vi "DATADYNTEST.vi"(8 "errin":errorcluster, 9 "SN":string="0B5MEVA000CA1JC1M0000041", 10 "Limites":T1, 11 "visain":refnum<visa-resource-name>) -> (0 "errout":errorcluster, 2 "chaîne concaténée":string, 3 "visaout":refnum<visa-resource-name>)   [LabVIEW 2020]
doc: "Test et trace en BDD l'OCV et les V/TCell"
uses:
  <vilib>/addons/database/Connection.llb/DB Tools Open Connec (String).vi
  <vilib>/addons/database/Connection.llb/Conn Execute.vi
  <vilib>/addons/database/Recordset.llb/Rec Destroy - Connection.vi
  <vilib>/addons/database/NI_Database_API.lvlib
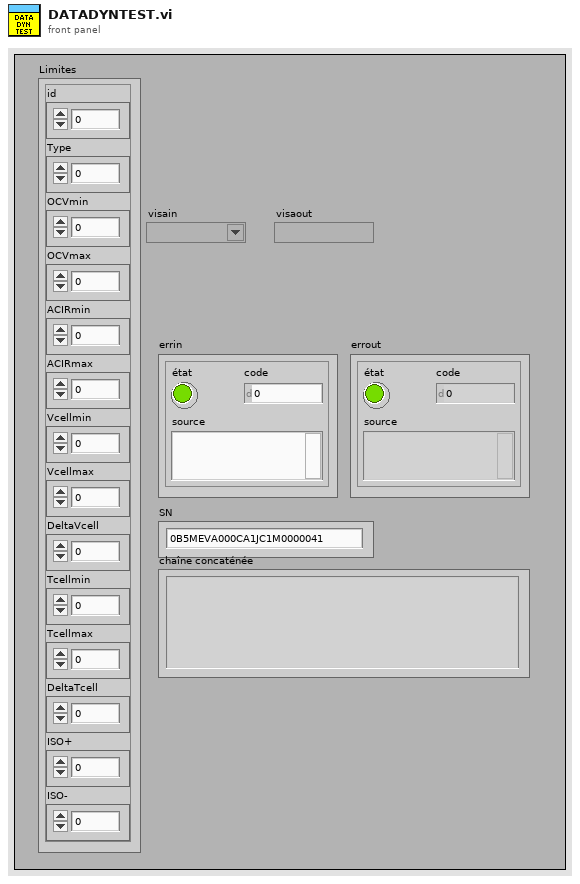
[diagram p1: front panel]
types:
  T1 = cluster{"id":dbl, "Type":dbl, "OCVmin":dbl, "OCVmax":dbl, "ACIRmin":dbl, "ACIRmax":dbl, "Vcellmin":dbl, "Vcellmax":dbl, "DeltaVcell":dbl, "Tcellmin":dbl, "Tcellmax":dbl, "DeltaTcell":dbl, "ISO+":dbl, "ISO-":dbl}
  T2 = cluster{"Cell1 V":sgl, "Cell2 V":sgl, "Cell3 V":sgl, "Cell4 V":sgl, "Cell1 °C":sgl, "Cell2 °C":sgl, "Cell5 V":sgl, "Cell6 V":sgl}
  T3 = typedef "NI_Database_API.lvlib/Conn ObjectReference.ctl" = refnum<k1>
  T4 = typedef "NI_Database_API.lvlib/Rec ObjectReference.ctl" = refnum<k1>
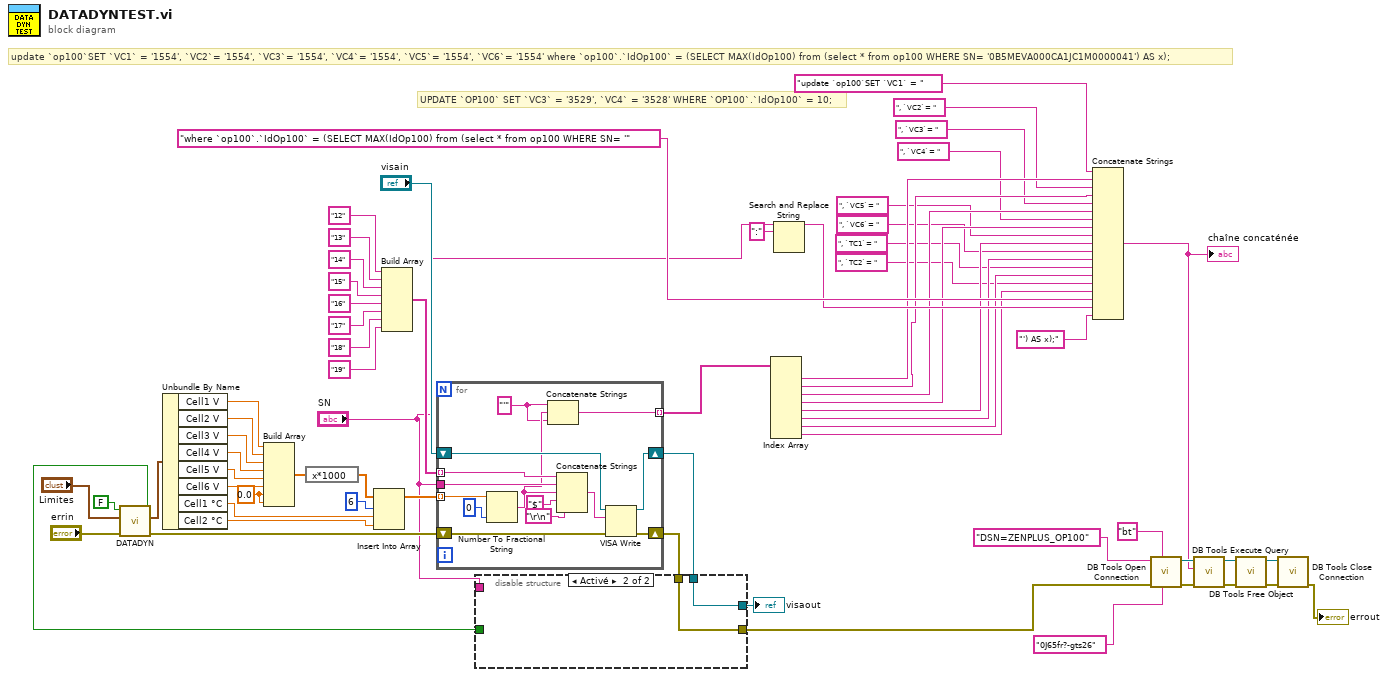
[diagram p0: block diagram]
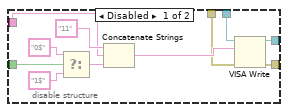
[diagram p2: hidden frame]
diagram:
  w39 = sgl 0.0 ("élément")
  # "update `op100`SET `VC1` = '1554', `VC2`= '1554', `VC3`= '1554', `VC4`= '1554', `VC5`= '1554', `VC6`= '1554' where `op100`.`IdOp100` = (SELECT MAX(IdOp100) from (select * from op100 WHERE SN= '0B5MEVA000CA1JC1M0000041') AS x);"
  # "UPDATE `OP100` SET `VC3` = '3529', `VC4` = '3528' WHERE `OP100`.`IdOp100` = 10;"
  n1 = call "DATADYN.vi"("errin"="errin", "Limites"="Limites", "3P4S"=FALSE) -> ("errout"=w64:errorcluster, "Out"=w42:T2, "test OK?"=w38:bool)  [unwired: 5 in, 1 out]
  n2 = Unbundle By Name(w42) -> ("Cell1 V"=w52:sgl, "Cell2 V"=w53:sgl, "Cell3 V"=w54:sgl, "Cell4 V"=w55:sgl, "Cell5 V"=w56:sgl, "Cell6 V"=w57:sgl, "Cell1 °C"=w61:sgl, "Cell2 °C"=w62:sgl)
  n3 = Build Array(w52, w53, w54, w55, w56, w57, w39, w39) -> (w58:sgl[])
  n4 = expression code="x*1000"(w58) -> (w59:sgl[])
  n5 = Insert Into Array(array=w59, index=6 ("indice"), new element #1=w61, new element #2=w62) -> (w63:sgl[])
  n6 = Build Array("12", "13", "14", "15", "16", "17", "18", "19") -> (w51:string[])
  n7 = for {
    tunnel: w51 -> [w80] mode=indexing
    tunnel: "SN" -> [w79]
    tunnel: w63 -> [w78] mode=indexing
    shift-right: [w71] -> w37
    shift-left: "visain" -> [w72]
    shift-right: [w73] -> w35
    shift-left: w64 -> [w75]
    tunnel: [w67] -> w20 mode=indexing
    w68 = "'" ("chaîne")
    n8 = Number To Fractional String ("Nombre en chaîne fractionnaire")(number=w78, precision (6)=i16 0 ("précision (6)")) -> (F-format string=w69:string)  [unwired: 2 in]
    n9 = Concatenate Strings(w68, w69, w68) -> (w67:string)
    n10 = Concatenate Strings(w80, w79, w69, "$" ("chaîne"), "\r\n") -> (w74:string)
    n11 = VISA Write(VISA resource name=w72, write buffer=w74, error in (no error)=w75) -> (VISA resource name out=w71:refnum<visa-resource-name>, error out=w73:errorcluster)  [unwired: 1 out]
  }
  n12 = disable-structure shown="Activé" {
    disable-tunnel: w38 -> [w87 _]
    disable-tunnel: "SN" -> [w86 _]
    disable-tunnel: w37 -> [w84 w93]
    disable-tunnel: [w83 w93] -> w36
    disable-tunnel: [w82 w92] -> w6
    disable-tunnel: w35 -> [w81 w92]
    frame Disabled {
      n13 = Select(t="0$" ("chaîne"), s=w87, f="1$" ("chaîne")) -> (s? t:f=w88:string)
      n14 = Concatenate Strings("11" ("chaîne"), w86, w88) -> (w85:string)
      n15 = VISA Write(VISA resource name=w84, write buffer=w85, error in (no error)=w81) -> (VISA resource name out=w83:refnum<visa-resource-name>, error out=w82:errorcluster)  [unwired: 1 out]
    }
    frame Enabled {
    }
  }
  "visaout" <- w36
  n16 = Index Array(array=w20) -> (element #1=w19:string, element #2=w17:string, element #3=w15:string, element #4=w13:string, element #5=w11:string, element #6=w9:string, element #7=w4:string, element #8=w1:string)  [unwired: 8 in]
  n17 = Search and Replace String ("Rechercher et remplacer une chaîne")(input string="SN", search string=":" ("chaîne recherchée")) -> (result string=w22:string)  [unwired: 6 in, 3 out]
  n18 = Concatenate Strings("update `op100`SET `VC1` = " ("chaîne"), w19, ", `VC2`= " ("chaîne"), w17, ", `VC3`= " ("chaîne"), w15, ", `VC4`= " ("chaîne"), w13, ", `VC5`= " ("chaîne"), w11, ", `VC6`= " ("chaîne"), w9, ", `TC1`= " ("chaîne"), w4, ", `TC2`= " ("chaîne"), w1, "where `op100`.`IdOp100` = (SELECT MAX(IdOp100) from (select * from op100 WHERE SN= '" ("chaîne"), w22, "') AS x);" ("chaîne")) -> (w29:string)
  "chaîne concaténée" <- w29
  n19 = call-poly <vilib>:"DB Tools Open Connection.vi"("password"="0J65fr?-gts26", "userID"="bt", "error in (no error)"=w6, "connection information"="DSN=ZENPLUS_OP100") -> ("error out"=w34:errorcluster, "connection reference"=w32:T3)  [unwired: 4 in]
  n20 = call-poly <vilib>:"DB Tools Execute Query.vi"("error in (no error)"=w34, "SQL query"=w29, "connection reference"=w32) -> ("error out"=w25:errorcluster, "recordset reference"=w24:T4)  [unwired: 5 in]
  n21 = call-poly <vilib>:"DB Tools Free Object.vi"("error in (no error)"=w25, "recordset reference"=w24) -> ("error out"=w33:errorcluster, "connection reference"=w31:T3)  [unwired: 8 in]
  n22 = call <vilib>:"DB Tools Close Connection.vi"("error in (no error)"=w33, "connection reference"=w31) -> ("error out"=→"errout":errorcluster)  [unwired: 5 in]
